vi "Target Prosthesis Angle Manager.vi"(8 "Prosthesis Side":enum16{"Right Foot", "Left Foot"}(ring), 11 "Encoder Angle (deg)":dbl) -> (3 "Prosthesis Angle (deg)":dbl)   [LabVIEW 2018, in "COBRA Measurement and Filtering Library.lvlib"]
uses:
  COBRA Measurement and Filtering Library.lvlib
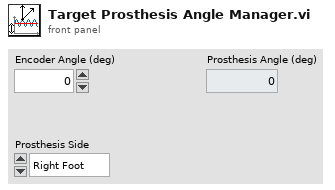
[diagram p1: front panel]
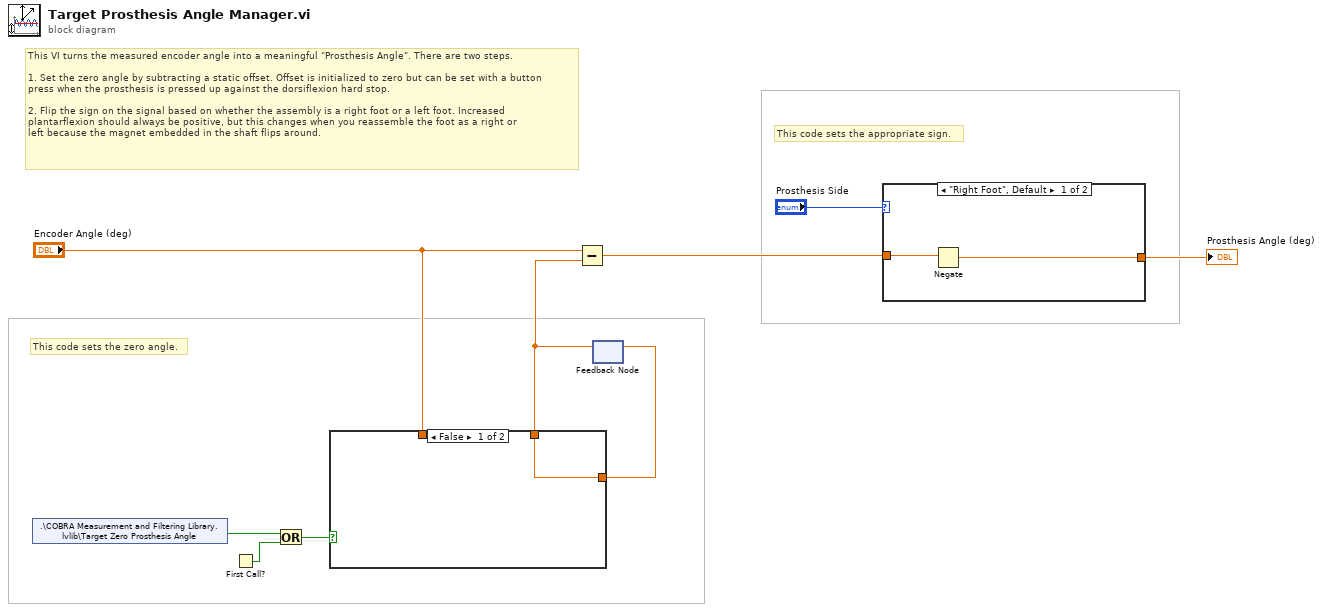
[diagram p0: block diagram]
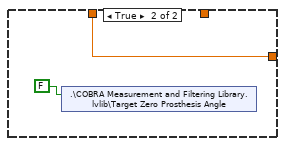
[diagram p3: hidden frame]
diagram:
  # "This code sets the appropriate sign."
  # "This code sets the zero angle."
  # "This VI turns the measured encoder angle into a meaningful \"Prosthesis Angle\". There are two steps.\n\n1. Set the zero angle by subtracting a static offset. Offset is initialized to zero but can be set with a button\npress when the prosthesis is pressed up against the dorsiflexion hard stop.\n\n2. Flip the sign on the signal based on whether the assembly is a right foot or a left foot. Increased \nplantarflexion should always be positive, but this changes when you reassemble the foot as a right or\nleft because the magnet embedded in the shaft flips around."
  n1 = shared-variable ".\\COBRA Measurement and Filtering Library.lvlib\\Target Zero Prosthesis Angle"() -> (w5:bool)  [unwired: 1 in, 1 out]
  n2 = First Call?() -> (First Call?: T/F=w7:bool)
  n3 = Or(x=w5, y=w7) -> (x .or. y?=w8:bool)
  n4 = feedback #1() -> (w6:dbl)  [unwired: 1 in]
  n5 = case shown="False" w8 {
    tunnel: "Encoder Angle (deg)" -> [_ w12]
    tunnel: [w10 w12] -> w9
    tunnel: w6 -> [w10 _]
    frame False {
    }
    frame True {
      n6 = shared-variable ".\\COBRA Measurement and Filtering Library.lvlib\\Target Zero Prosthesis Angle"(FALSE ("PXI Zero Prosthesis Angle")) -> ()  [unwired: 1 in, 1 out]
    }
  }
  n7 = Subtract(x="Encoder Angle (deg)", y=w6) -> (x-y=w3:dbl)
  n8 = feedback-in #1(w9) -> ()
  n9 = case shown="\"Right Foot\", Default" "Prosthesis Side" {
    tunnel: w3 -> [w14 w15]
    tunnel: [w13 w15] -> w1
    frame "Right Foot", Default {
      n10 = Negate(x=w14) -> (-x=w13:dbl)
    }
    frame "Left Foot" {
    }
  }
  "Prosthesis Angle (deg)" <- w1
